vi "RDS Child Write Subscribed IDs.vi"(8 "error in (no error)":errorcluster, 10 "Subscribed IDs":T1[](array[typedef]), 11 "RDS Parent Actor in":refnum<class "RDS Parent Actor.lvclass">) -> (0 "error out":errorcluster, 3 "RDS Parent Actor out":refnum<class "RDS Parent Actor.lvclass">)   [LabVIEW 2015, in "RDS Abstracts.lvlib" / "RDS Parent Actor.lvlib" / "RDS Parent Actor.lvclass"]
uses:
  RDS Parent Actor.lvclass
  Libraries/RDS Framework/RDS Message ID.ctl
  RDS Parent Actor.lvclass/RDS Parent Actor.ctl
  Libraries/RDS Child Messages/RDS Child Messages.lvlib
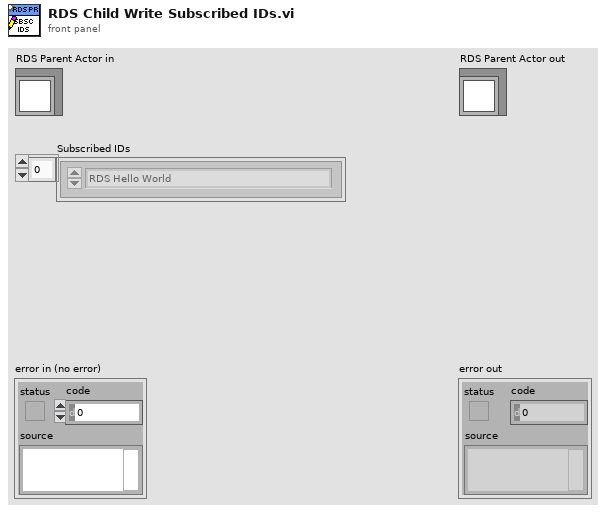
[diagram p1: front panel]
types:
  T1 = typedef "RDS Child Messages.lvlib/RDS Message ID.ctl" = enum16{"RDS Hello World", "String Message", "AIP_Status", "AIP_Command", "GPS_Data", "MCB_Command", "MCB_Status", "Compass_Data", "Depth_Data", "Battery_Data", "Contoller_State", "Set_Mag_Dev", "BTB_Shutdown", "State_Sample_Request", "State_Sample", "PID_Gains_Set", "Helm_Limiter_Set", "Helm_Heading_Command", "Helm_Steering_Command", "Helm_Status", "Controller_Message", "AIP_Set_Min_Depth", "Mission_Controller_State", "Mission_Upload", "Mission_Set_Op_and_Run", "Mission_Settings_Set"}
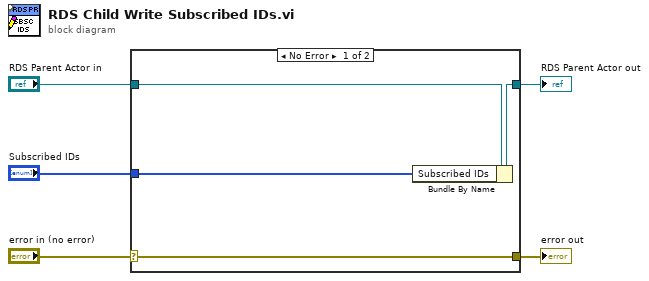
[diagram p0: block diagram]
diagram:
  n1 = case shown="No Error" "error in (no error)" {
    selector: "error in (no error)" -> [w9 w10]
    tunnel: [w9 w10] -> w4
    tunnel: [w7 w11] -> w2
    tunnel: "RDS Parent Actor in" -> [w8 w11]
    tunnel: "Subscribed IDs" -> [w6 _]
    frame No Error {
      n2 = Bundle By Name(cluster=w8, "Subscribed IDs"=w6) -> (w7:refnum<class "RDS Parent Actor.lvclass">)
    }
    frame Error {
    }
  }
  "error out" <- w4
  "RDS Parent Actor out" <- w2
